vi "gainCompression.vi"(8 "compressionMin":dbl=-6.0 format="%#_13g", 10 "slaveInput":dbl format="%#_6p", 11 "masterInput":dbl format="%#_6p") -> (0 "gainScale":i8, 2 "rescaledSlave":fxp<+/-,20,1> format="%#_6p", 3 "rescaledMaster":fxp<+/-,20,1> format="%#_6p")   [LabVIEW 2016]
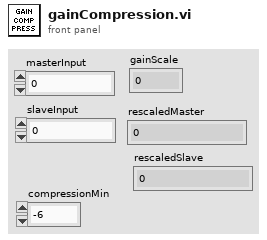
[diagram p1: front panel]
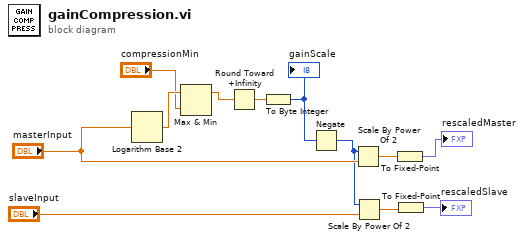
[diagram p0: block diagram]
diagram:
  n1 = Logarithm Base 2(1:"masterInput") -> (0:w9:dbl)
  n2 = Max & Min(x=w9, y="compressionMin") -> (max(x,y)=w7:dbl)  [unwired: 1 out]
  n3 = Round Toward +Infinity(x=w7) -> (ceil(x): smallest int >= x=w5:dbl)
  n4 = To Byte Integer(number=w5) -> (8bit integer=w4:i8)
  "gainScale" <- w4
  n5 = Negate(x=w4) -> (-x=w2:i8)
  n6 = Scale By Power Of 2(n=w2, x="masterInput") -> (x*2^n=w12:dbl)
  n7 = Scale By Power Of 2(n=w2, x="slaveInput") -> (x*2^n=w3:dbl)
  n8 = To Fixed-Point(number=w12) -> (fixed-point=→"rescaledMaster":fxp<+/-,20,1>)  [unwired: 1 in]
  n9 = To Fixed-Point(number=w3) -> (fixed-point=→"rescaledSlave":fxp<+/-,20,1>)  [unwired: 1 in]
